vi "Create_RFID_Baseband smallQuery.vi"(5 "Parameters Symbols":T3={"Tari"=8e-06, "PW"=0.5, "factor for \"1\" symbol"=0.5, "RTcal"=2.5, "TRcal"=3.0, "Delimiter"=1.25e-05} {"TRcal" min=1.1 max=3.0 step=0.1; "RTcal" min=2.5 max=3.0 step=0.1; "factor for \"1\" symbol" min=0.5 max=1.0 step=0.1; "PW" min=0.265 max=0.525 step=0.001; "Tari" format="%#_3p"}, 9 "Symbol Rate [Hz]":dbl, 11 "error in":errorcluster, 12 "Parameters Query":T1={"DR"=FALSE, "M"=1, "TRext (T=Pilot Tone)"=FALSE, "Sel"=1, "Session"=0, "Q"=0, "Target"=FALSE} {"Session" items=["S0", "S1", "S2", "S3"]; "Sel" items=["All", "All2", "~SL", "SL"]; "M" items=["M=1", "M=2", "M=4", "M=8"]}) -> (6 "complex waveform":cluster{"t0":dbl, "dt":dbl, "Y":cdb[]}, 15 "error out":errorcluster)   [LabVIEW 2015]
uses:
  <vilib>/addons/Modulation/Analog/support/mod_Set Error Source.vi
  <vilib>/addons/Modulation/Digital/General/MT Generate ASK system parameters (M).vi
  <vilib>/addons/Modulation/Digital/Support/Common/Validators/mod_Generate Filter Coefficients Validate.vi
  <vilib>/addons/Modulation/Digital/General/subVIs/mod_Generate Filter Coefficients.vi
  <vilib>/addons/Modulation/niDMT.lvlib
panel:
  out "ASK system parameters":T2 {"symbol map" format="%.3f"}
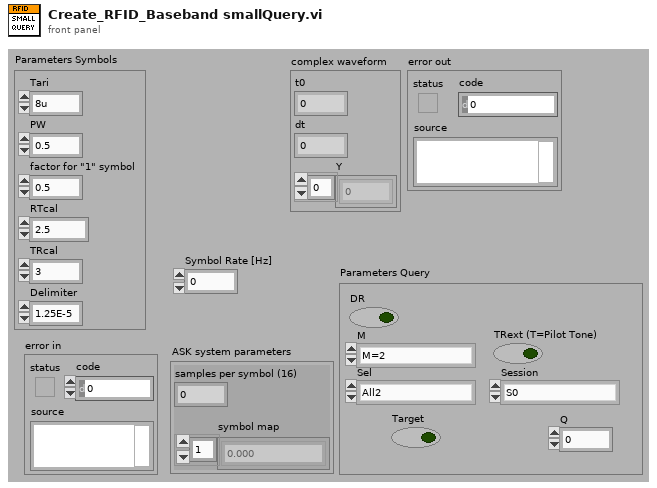
[diagram p1: front panel]
types:
  T1 = cluster{"DR":bool, "M":u16, "TRext (T=Pilot Tone)":bool, "Sel":u16, "Session":u16, "Q":u8, "Target":bool}
  T2 = cluster{"samples per symbol (16)":i32, "symbol map":cdb[]}
  T3 = cluster{"Tari":dbl, "PW":dbl, "factor for \"1\" symbol":dbl, "RTcal":dbl, "TRcal":dbl, "Delimiter":dbl}
  T4 = enum16{"none", "Raised Cosine", "Root Raised Cos", "Gaussian"}
  T5 = typedef "niAMT.lvlib/Complex Data Waveform.ctl" = cluster{"t0":dbl, "dt":dbl, "Y":cdb[]}
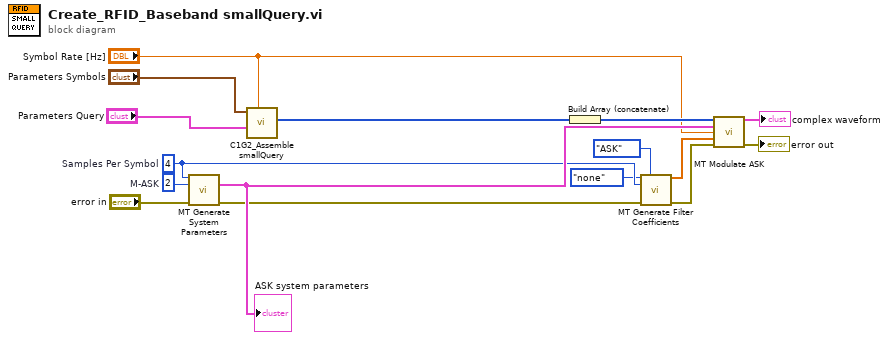
[diagram p0: block diagram]
diagram:
  w11 = 2  # M-ASK
  w7 = 4  # Samples Per Symbol
  n1 = call-poly <vilib>:"MT Generate System Parameters.vi"("samples per symbol (16)"=w7, "M-ASK (2)"=w11, "error in (no error)"="error in") -> ("ASK system parameters"=w12:T2, "error out"=w9:errorcluster)  [unwired: 10 in, 1 out]
  "ASK system parameters" <- w12
  n2 = call "C1G2_Assemble smallQuery.vi"("Symbol Rate"="Symbol Rate [Hz]", "Parameters Query"="Parameters Query", "Parameters Symbols"="Parameters Symbols") -> ("Signal out"=w4:u8[])  [unwired: 8 in]
  n3 = Build Array (concatenate)(w4) -> (w5:u8[])
  n4 = call <vilib>:"MT Generate Filter Coefficients.vi"("pulse shaping filter (none)"=T4."none", "modulation type"=enum16{"FSK", "PSK", "QAM", "MSK", "PAM", "ASK"}."ASK", "pulse shaping samples per symbol (16)"=w7, "error in (no error)"=w9) -> ("pulse shaping filter coefficients"=w13:dbl[], "error out"=w8:errorcluster)  [unwired: 9 in, 1 out]
  n5 = call <vilib>:"MT Modulate ASK.vi"("input bit stream"=w5, "ASK system parameters"=w12, "symbol rate (Hz)"="Symbol Rate [Hz]", "pulse shaping filter coefficients"=w13, "error in (no error)"=w8) -> ("output complex waveform"=→"complex waveform":T5, "error out"=→"error out":errorcluster)  [unwired: 8 in, 1 out]
